vi "FT_Close_Device.vi"(1 "Handle":u64) -> (0 "FT_Status":u64)   [LabVIEW 2017]
uses:
  Windows/System32/DriverStore/FileRepository/ftdibus.inf_amd64_49b3e24305b20ada/amd64/ftd2xx64.dll
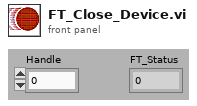
[diagram p1: front panel]
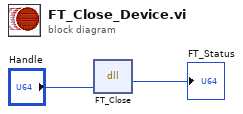
[diagram p0: block diagram]
diagram:
  n1 = dll-call lib="C:/Windows/System32/DriverStore/FileRepository/ftdibus.inf_amd64_49b3e24305b20ada/amd64/ftd2xx64.dll" fn="FT_Close"("Handle"="Handle") -> ("FT_Status"=→"FT_Status":u64)  [unwired: 4 in, 2 out]
